vi "Apply_Power_Control_Setpoints_14.vi"(0 "SI804.lvclass in":refnum<class "SI804.lvclass">, 1 "3 JSA60 DX811 XA01":bool, 2 "3 JSA60 DX812 XA01":bool, 3 "3 JSA10 FT112 XA01":bool, 5 "error in":errorcluster) -> (14 "SI804.lvclass out":refnum<class "SI804.lvclass">, 15 "Apply NFL SP":bool, 16 "Apply NFL Grad":bool, 17 "Apply ACT SP":bool, 19 "error out":errorcluster)   [LabVIEW 2022 SP3, in "SI804.lvclass"]
uses:
  SI804.lvclass
  SI804.lvclass/SI804.ctl
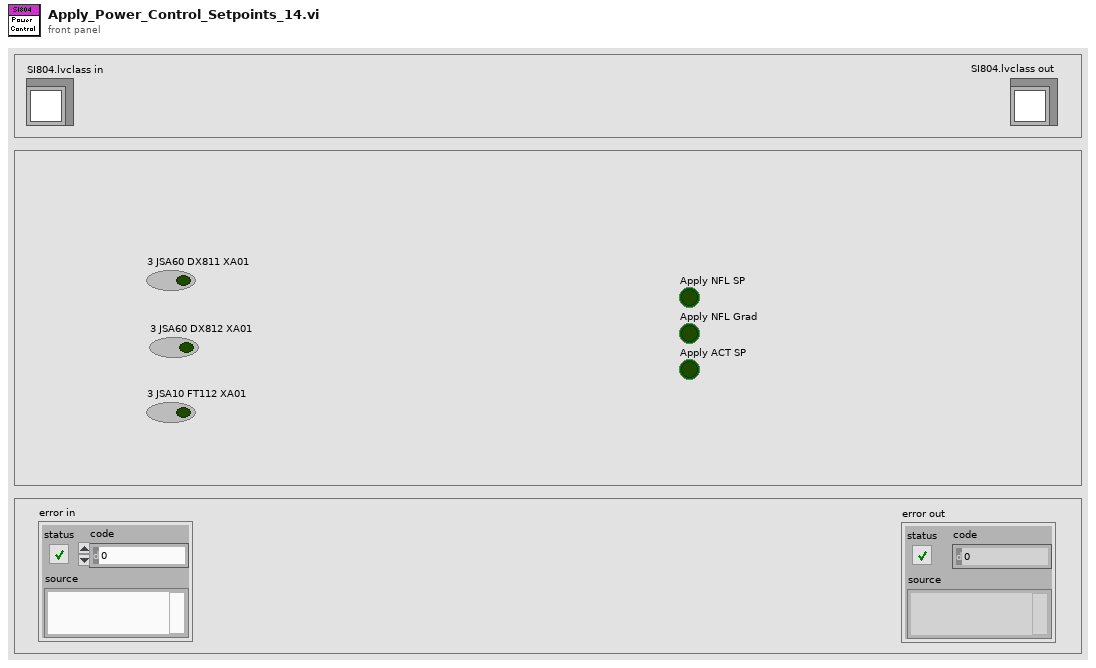
[diagram p1: front panel]
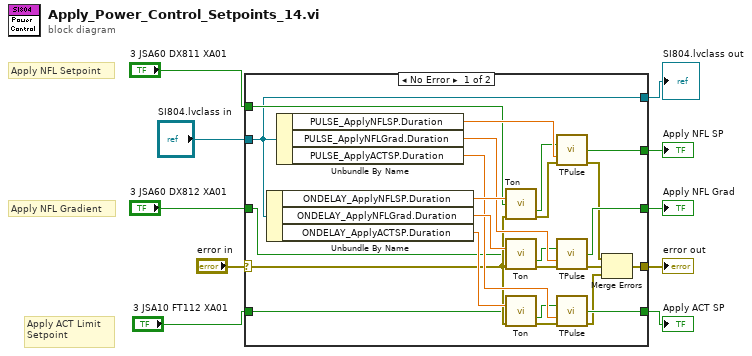
[diagram p0: block diagram]
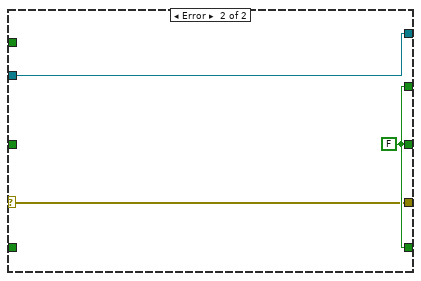
[diagram p2: hidden frame]
diagram:
  # "Apply ACT Limit\nSetpoint"
  # "Apply NFL Gradient"
  # "Apply NFL Setpoint"
  n1 = case shown="No Error" "error in" {
    selector: "error in" -> [w28 w36]
    tunnel: "3 JSA60 DX811 XA01" -> [w21 _]
    tunnel: "3 JSA60 DX812 XA01" -> [w20 _]
    tunnel: "3 JSA10 FT112 XA01" -> [w19 _]
    tunnel: "SI804.lvclass in" -> [w11 w35]
    tunnel: [w18 w37] -> w5
    tunnel: [w17 w37] -> w4
    tunnel: [w16 w37] -> w3
    tunnel: [w12 w36] -> w2
    tunnel: [w11 w35] -> w1
    frame No Error {
      n2 = Unbundle By Name(w11) -> ("ONDELAY_ApplyNFLSP.Duration"=w34:dbl, "ONDELAY_ApplyNFLGrad.Duration"=w33:dbl, "ONDELAY_ApplyACTSP.Duration"=w32:dbl)
      n3 = Unbundle By Name(w11) -> ("PULSE_ApplyNFLSP.Duration"=w31:dbl, "PULSE_ApplyNFLGrad.Duration"=w30:dbl, "PULSE_ApplyACTSP.Duration"=w29:dbl)
      n4 = call "Ton.vi"("Ton"=w34, "input"=w21, "error in"=w28) -> ("Binary out"=w24:bool, "error out"=w27:errorcluster)  [unwired: 8 in, 3 out]
      n5 = call "Ton.vi"("Ton"=w33, "input"=w20, "error in"=w28) -> ("Binary out"=w23:bool, "error out"=w26:errorcluster)  [unwired: 8 in, 3 out]
      n6 = call "Ton.vi"("Ton"=w32, "input"=w19, "error in"=w28) -> ("Binary out"=w22:bool, "error out"=w25:errorcluster)  [unwired: 8 in, 3 out]
      n7 = call "TPulse.vi"("trigger"=w24, "TPulse"=w31, "error in"=w27) -> ("output"=w18:bool, "error out"=w15:errorcluster)  [unwired: 10 in, 1 out]
      n8 = call "TPulse.vi"("trigger"=w23, "TPulse"=w30, "error in"=w26) -> ("output"=w17:bool, "error out"=w14:errorcluster)  [unwired: 10 in, 1 out]
      n9 = call "TPulse.vi"("trigger"=w22, "TPulse"=w29, "error in"=w25) -> ("output"=w16:bool, "error out"=w13:errorcluster)  [unwired: 10 in, 1 out]
      n10 = Merge Errors(w15, w14, w13) -> (w12:errorcluster)
    }
    frame Error {
      w37 = FALSE ("output")
    }
  }
  "Apply NFL SP" <- w5
  "Apply NFL Grad" <- w4
  "Apply ACT SP" <- w3
  "error out" <- w2
  "SI804.lvclass out" <- w1
